vi "IncStepsESP.vi"(0 "ESP VISA IN":refnum<visa-resource-name>, 1 "Digitizer Settings":T9={"Digitizer delay (us) "=0.0, "rf points per line"=2048, "lines per plane"=128, "Samp Rate (Hz)"=100000000.0, "Additional dig delay (us)"=0.0, "Voltage Scale"=0.4, "Pre-Looks"=0, "Offset delay (us)"=0.0, "bits A/D"=8, "Avg Num"=1, "DigTimeOut"=5.0, "Rel Dig Delay"=0.0, "Dig Ch"=0, "LeCroyCluster"={"LeCroy Channels"=[TRUE, FALSE, FALSE, FALSE], "LC read pt offset"=0.0, "Sweep Avg"=FALSE}, "Main Digitizer"=enum."NI Digitizer", "Dig Config"=enum."Single channel", "Digitizer ID Cluster"={"Acqiris/Alazar/SP ID"=[], "NI Instr Handles"=[], "LeCroy VISA"="", "GaGe Handle"={"Handle"=0, "Sample size"=0, "Resolution"=0, "Offset"=0, "Channels"=0, "Boards"=0}, "ATS Ref"="ATS9350", "Acqiris Address"=["PCI::INSTR0"], "ADQRef"=refnum, "adq_cu_ptr"=refnum}, "Trigger Settings"={"Trig Source"=1, "Trig Coupling"=0, "Trig Slope"=0, "Level (mV)"=1500.0}, "Bulk Acq"=FALSE, "Bulk Start Indexes"=[], "Data Ref RF"=refnum, "NI ID/Channel"=[], "Total Dig CH"=1, "Xtra Ann Trig delay (us)"=10.0, "Fix Z Delay?"=FALSE, "One Way Transmission?"=FALSE, "Data Ref Log"=refnum} {"Trigger Settings"."Trig Slope" items=["Positive", "Negative"]; "Trigger Settings"."Level (mV)" format="%.2f"; "Trigger Settings"."Trig Coupling" items=["DC 1 MOhm", "AC 1 MOhm", "DC 50 Ohm", "AC 50 Ohm"]; "Trigger Settings"."Trig Source" items=["Chan 1", "External"]; "Rel Dig Delay" format="%.2f"; "DigTimeOut" format="%.2f"; "Avg Num" min=1; "Offset delay (us)" format="%.2f"; "Additional dig delay (us)" format="%.2f"; "Digitizer delay (us)" format="%.2f"}, 2 "Ann Array Params":T2={"Synth Foc?"=FALSE, "Focal Zones"=41, "Switch T/R"=0, "Trans Geometry (mm)"={"Transducer"=0, "Geo Focus"=12.0, "a (radius)"=3.0, "# of rings"=5, "kerf space "=0.1, "Center Freq"=12.0}, "Sub Ap Excite?"=FALSE, "Full Array Scan?"=FALSE, "Xmt/Rcv"={"XMIT"=[TRUE, TRUE, TRUE, TRUE, TRUE], "RCV"=[TRUE, TRUE, TRUE, TRUE, TRUE]}, "PulseSpacing (us)"=0.0, "Xmit Ring"=0, "XMIT CHS"=0, "RCV CHS"=0, "GPU?"=FALSE, "Save TIFF?"=FALSE, "downfactor"=1, "RCV 1CH"=0} {"RCV 1CH" items=["All", "1", "2", "3", "4", "5"]; "Trans Geometry (mm)"."Transducer" items=["6D 12R 40 MHz"=0, "10D 31R 20 MHz"=1, "10D 23R 20 MHz"=2, "6D 23R 40 MHz"=3, "4.5D 10.7R 40 MHz"=4, "9D 23.5R 20 MHz"=5, "9D 25.8R 20MHz"=6, "Enter"=99]; "Switch T/R" min=1 max=5 step=1}, 3 "Avg Num":i32=1, 5 "number of scans":i32=128, 7 "Motion Settings":T5={"No Motion?"=FALSE, "Motion System"=enum."NI 735x", "Motion Bd ID"=1, "Motion Profile"="SMAC1", "# Axis"=1, "Reverse Z axis?"=TRUE, "SMAC Axis"=0, "scan pair"=enum."y-(x) scan", "RT fps"=6.0, "Steps per mm"=[1000, 1000, 1000, 1000], "Motor Parameters"={"velocity ct/s"=[10000.0, 10000.0, 10000.0, 50000.0], "accel ct/s^2"=[50000.0, 50000.0, 50000.0, 200000.0]}, "One Way Scan"=FALSE, "Reverse One Way Scan"=FALSE, "Global Position (mm)"=[], "Plane"=0, "Distance between\nscan lines (um)"=0.0, "Distance between\nscan planes (um)"=0.0, "number of scan planes"=1, "Total steps in line"=0, "Xtra plane\ndistance  (um)"=100, "Xtra planes "=1, "Add Axis"=FALSE, "overshoot cts"=200, "BKPT Shift"=0, "Scan Start Time (ms)"=0, "ESP VISA"="GPIB::1::INSTR", "3rd Axis"=1, "GL Ref Out"=refnum, "Galil Address"=""} {"3rd Axis" items=["x", "y", "z", "w"]; "Xtra planes" min=1; "Xtra plane\ndistance  (um)" min=0; "Distance between\nscan planes (um)" format="%.2f"; "Distance between\nscan lines (um)" format="%.2f"; "SMAC Axis" items=["None"=0, "Axis 1"=1, "Axis 2"=2, "Axis 3"=3, "Axis 4"=4, "Axis 5"=5, "Axis 6"=6, "Axis 7"=7, "Axis 8"=8, "Vector Space 1"=17, "Vector Space 2"=18, "Vector Space 3"=19, "Vector Space 4"=20]; "Motion Bd ID" min=1 max=32 step=1}, 9 "Axis":i32=1 min=1 max=4, 11 "File Names":string[](array[string]), 12 "motion error in":errorcluster, 13 "Type of scan":T1, 14 "Reverse ?":bool) -> (4 "ESP VISA OUT":refnum<visa-resource-name>, 15 "Motion error":bool)   [LabVIEW 2022 SP3]
uses:
  Digitizers/-DigitizerRoutines/DigitizerSettings.ctl
  Digitizers/-DigitizerRoutines/Digitizer.ctl
  Digitizers/-DigitizerRoutines/DigConfig.ctl
  Digitizers/-DigitizerRoutines/DigitizerID.ctl
  C:/Windows/System32/ADQAPI_dotNet_helper.dll
  NI_controller/-NI_MotionRoutines/MotionParameters.ctl
  NI_controller/-NI_MotionRoutines/MotionSys.ctl
  -MotionRoutines/ScanAxis.ctl
  -MotionRoutines/3rdAxis.ctl
  Annular Array/-AnnularRoutines/AnnularArray.ctl
  Annular Array/-AnnularRoutines/TransGeometry.ctl
  Annular Array/-AnnularRoutines/ArrayGeometry.ctl
  -ScanSystem/Controls/ScanType2.ctl
  Galil/Command Menu.ctl
  <vilib>/Analysis/baseanly.llb/Mean (DBL).vi
  -MotionRoutines/MotionGlobals.vi
  <instrlib>/Acqiris Dx/Acqiris Dx.lvlib
  <instrlib>/Newport ESP301/Newport ESP301.lvlib
  <vilib>/Analysis/NI_AALBase.lvlib
panel:
  out "Intensity Graph":i16[][](graph)
  in  "Acq error in":errorcluster
  # "1-D and 2-D B scan settings"
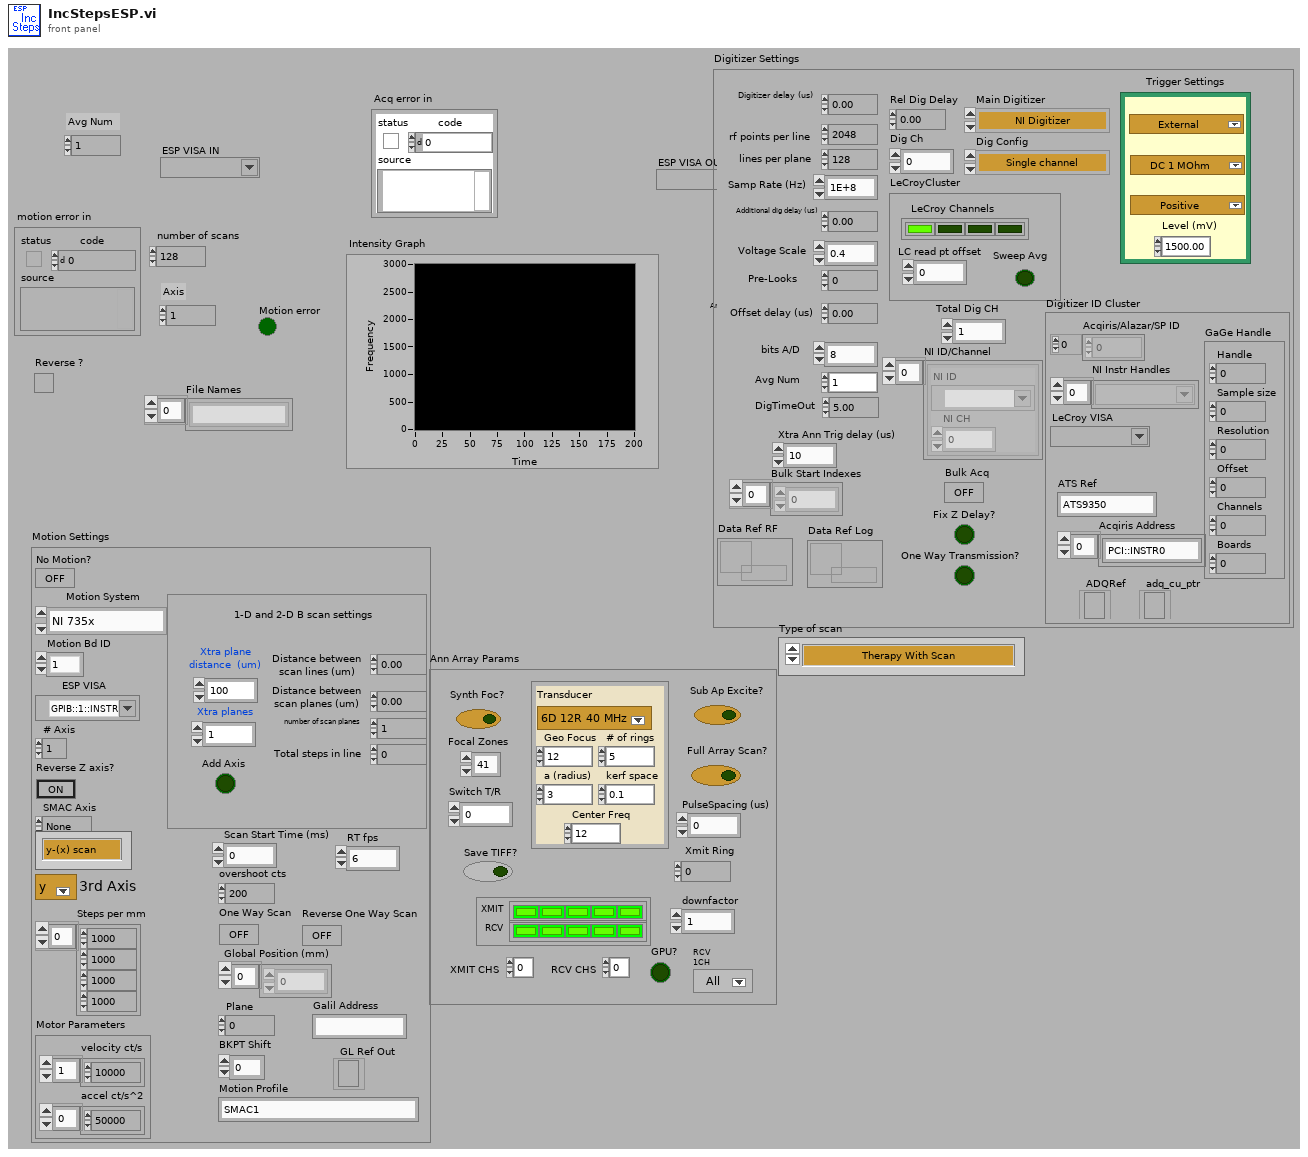
[diagram p1: front panel]
types:
  T1 = typedef "ScanType2.ctl" = enum16{"Therapy With Scan", "M scan", "M Scan With Therapy Burst", "1-D B Scan", "1-D B Scan With Therapy Burst", "2-D B Scan", "2-D B Scan With Therapy Burst", "Rotational Scan", "1-D B-Scan PRF", "2-D B-Scan PRF", "Real-Time Scan", "Contrast Agents", "1-D w/ Real-Time Set Up", "Dual Transducer", "Acoustic Microscopy", "Hydrophone Scanning"}
  T2 = typedef "AnnularArray.ctl" = cluster{"Synth Foc?":bool, "Focal Zones":i16, "Switch T/R":i16, "Trans Geometry (mm)":T3, "Sub Ap Excite?":bool, "Full Array Scan?":bool, "Xmt/Rcv":cluster{"XMIT":bool[], "RCV":bool[]}, "PulseSpacing (us)":sgl, "Xmit Ring":i32, "XMIT CHS":u8, "RCV CHS":u8, "GPU?":bool, "Save TIFF?":bool, "downfactor":i32, "RCV 1CH":u16}
  T3 = typedef "TransGeometry.ctl" = cluster{"Transducer":T4, "Geo Focus":dbl, "a (radius)":dbl, "# of rings":i32, "kerf space ":dbl, "Center Freq":dbl}
  T4 = typedef "ArrayGeometry.ctl" = u16
  T5 = typedef "MotionParameters.ctl" = cluster{"No Motion?":bool, "Motion System":T6, "Motion Bd ID":u8, "Motion Profile":string, "# Axis":i8, "Reverse Z axis?":bool, "SMAC Axis":u16, "scan pair":T7, "RT fps":sgl, "Steps per mm":i32[], "Motor Parameters":cluster{"velocity ct/s":dbl[], "accel ct/s^2":dbl[]}, "One Way Scan":bool, "Reverse One Way Scan":bool, "Global Position (mm)":dbl[], "Plane":i32, "Distance between\nscan lines (um)":sgl, "Distance between\nscan planes (um)":sgl, "number of scan planes":i32, "Total steps in line":i32, "Xtra plane\ndistance  (um)":i32, "Xtra planes ":i32, "Add Axis":bool, "overshoot cts":i32, "BKPT Shift":i32, "Scan Start Time (ms)":u32, "ESP VISA":refnum<visa-resource-name>, "3rd Axis":T8, "GL Ref Out":refnum<k7>, "Galil Address":string}
  T6 = typedef "MotionSys.ctl" = enum16{"MM3000", "NI 735x", "Newport ESP", "No Motion Card", "Galil"}
  T7 = typedef "ScanAxis.ctl" = enum16{"y-(x) scan", "x-(y) scan", "z-(x) scan", "z-(y) scan", "y-(z) scan", "x-(z) scan", "w-(x) scan", "w-(y) scan", "w-(z) scan", "x-(w) scan", "y-(w) scan", "z-(w) scan"}
  T8 = typedef "3rdAxis.ctl" = u16
  T9 = typedef "DigitizerSettings.ctl" = cluster{"Digitizer delay (us) ":dbl, "rf points per line":i32, "lines per plane":i32, "Samp Rate (Hz)":dbl, "Additional dig delay (us)":dbl, "Voltage Scale":dbl, "Pre-Looks":i32, "Offset delay (us)":dbl, "bits A/D":i8, "Avg Num":i32, "DigTimeOut":sgl, "Rel Dig Delay":sgl, "Dig Ch":i32, "LeCroyCluster":cluster{"LeCroy Channels":bool[], "LC read pt offset":dbl, "Sweep Avg":bool}, "Main Digitizer":T10, "Dig Config":T11, "Digitizer ID Cluster":T12, "Trigger Settings":cluster{"Trig Source":u16, "Trig Coupling":u16, "Trig Slope":u16, "Level (mV)":dbl}, "Bulk Acq":bool, "Bulk Start Indexes":i32[], "Data Ref RF":refnum<data-value>, "NI ID/Channel":cluster{"NI ID":refnum<k15>, "NI CH":i32}[], "Total Dig CH":i32, "Xtra Ann Trig delay (us)":dbl, "Fix Z Delay?":bool, "One Way Transmission?":bool, "Data Ref Log":refnum<data-value>}
  T10 = typedef "Digitizer.ctl" = enum16{"Acqiris Digitizer", "NI Digitizer", "LeCroy", "GaGe", "AlazarTech", "No Digitizer", "Teledyne"}
  T11 = typedef "DigConfig.ctl" = enum16{"Single channel", "2 Chans w/ 2 Acqiris", "2 Chans w/ 1 Acqiris", "5-CH Pulser New", "5-CH pulser w/ ann array", "5-pass style ann array", "Empty"}
  T12 = typedef "DigitizerID.ctl" = cluster{"Acqiris/Alazar/SP ID":u32[], "NI Instr Handles":refnum<k15>[], "LeCroy VISA":refnum<visa-resource-name>, "GaGe Handle":cluster{"Handle":u32, "Sample size":u32, "Resolution":i32, "Offset":i32, "Channels":u32, "Boards":u32}, "ATS Ref":string, "Acqiris Address":string[], "ADQRef":refnum<k24>, "adq_cu_ptr":refnum<k24>}
  T13 = typedef "location.ctl" = enum16{"Automatic", "WCM Main", "Hawaii", "Columbia MM3000", "Columbia  NI System", "NYU", "RRI 2", "UHI Allen", "CUMC RT", "Chiba", "Stony Brook", "WCM Microscopy", "WCM Aeoretch", "WCM Optics Lab", "WCM Main 2Axis", "WCM Rotation", "WCM SAM SMAC", "SERI GP"}
  T14 = typedef "Command Menu.ctl" = enum16{"CommandPassThrough", "Abort Motion", "Define Pos", "Velocity", "Acceleration", "Deceleration", "Position Rel", "Postion Abs", "Begin Move", "After Move", "Home", "KI", "KD", "KP", "IL", "Config I/O", "Set Bit", "Clear Bit", "Motor Off", "Moto On", "Status", "Execute", "Halt Execute", "HX Status", "Tell Velocity", "Check Motion", "BreakPoint", "Tell Position", "Current Code Line", "Tell Switches", "OC Force On", "OC Off", "Pos Soft Limit", "Rev Soft Limit"}
  T15 = cluster{"axis 1 +hardware travel limit":bool, "axis 2 +hardware travel limit ":bool, "axis 3 +hardware travel limit ":bool, "axis 4 +hardware travel limit ":bool, "axis 5 +hardware travel limit ":bool, "axis 6 +hardware travel limit ":bool, "reserved":bool, "reserved":bool, "axis 1 -hardware travel limit ":bool, "axis 2 -hardware travel limit ":bool, "axis 3 -hardware travel limit ":bool, "axis 4 -hardware travel limit ":bool, "axis 5 -hardware travel limit ":bool, "axis 6 -hardware travel limit ":bool, "reserved":bool, "reserved":bool, "axis 1 amplifier fault input":bool, "axis 2 amplifier fault input":bool, "axis 3 amplifier fault input":bool, "axis 4 amplifier fault input":bool, "axis 5 amplifier fault input":bool, "axis 6 amplifier fault input":bool, "reserved":bool, "reserved":bool, "reserved":bool, "reserved":bool, "reserved":bool, "100-pin emergency stop (unlatched) low":bool, "auxiliary I/O emergency stop (latched)":bool, "100-pin connector emergency stop (latched)":bool, "auxiliary I/O connector emergency stop (latched)":bool, "100-pin cable interlock":bool}
  T16 = cluster{"Port A bit-0 at logic level":bool, "Port A bit-1 at logic level":bool, "Port A bit-2 at logic level ":bool, "Port A bit-3 at logic level":bool, "Port A bit-4 at logic level":bool, "Port A bit-5 at logic level ":bool, "Port A bit-6 at logic level ":bool, "Port A bit-7 at logic level ":bool, "Port B bit-0 at logic level":bool, "Port B bit-1 at logic level":bool, "Port B bit-2 at logic level ":bool, "Port B bit-3 at logic level":bool, "Port B bit-4 at logic level":bool, "Port B bit-5 at logic level ":bool, "Port B bit-6 at logic level ":bool, "Port B bit-7 at logic level ":bool}
  T17 = cluster{sgl, "Gain [dB]  ":sgl, "Atten (dB)":sgl}[]
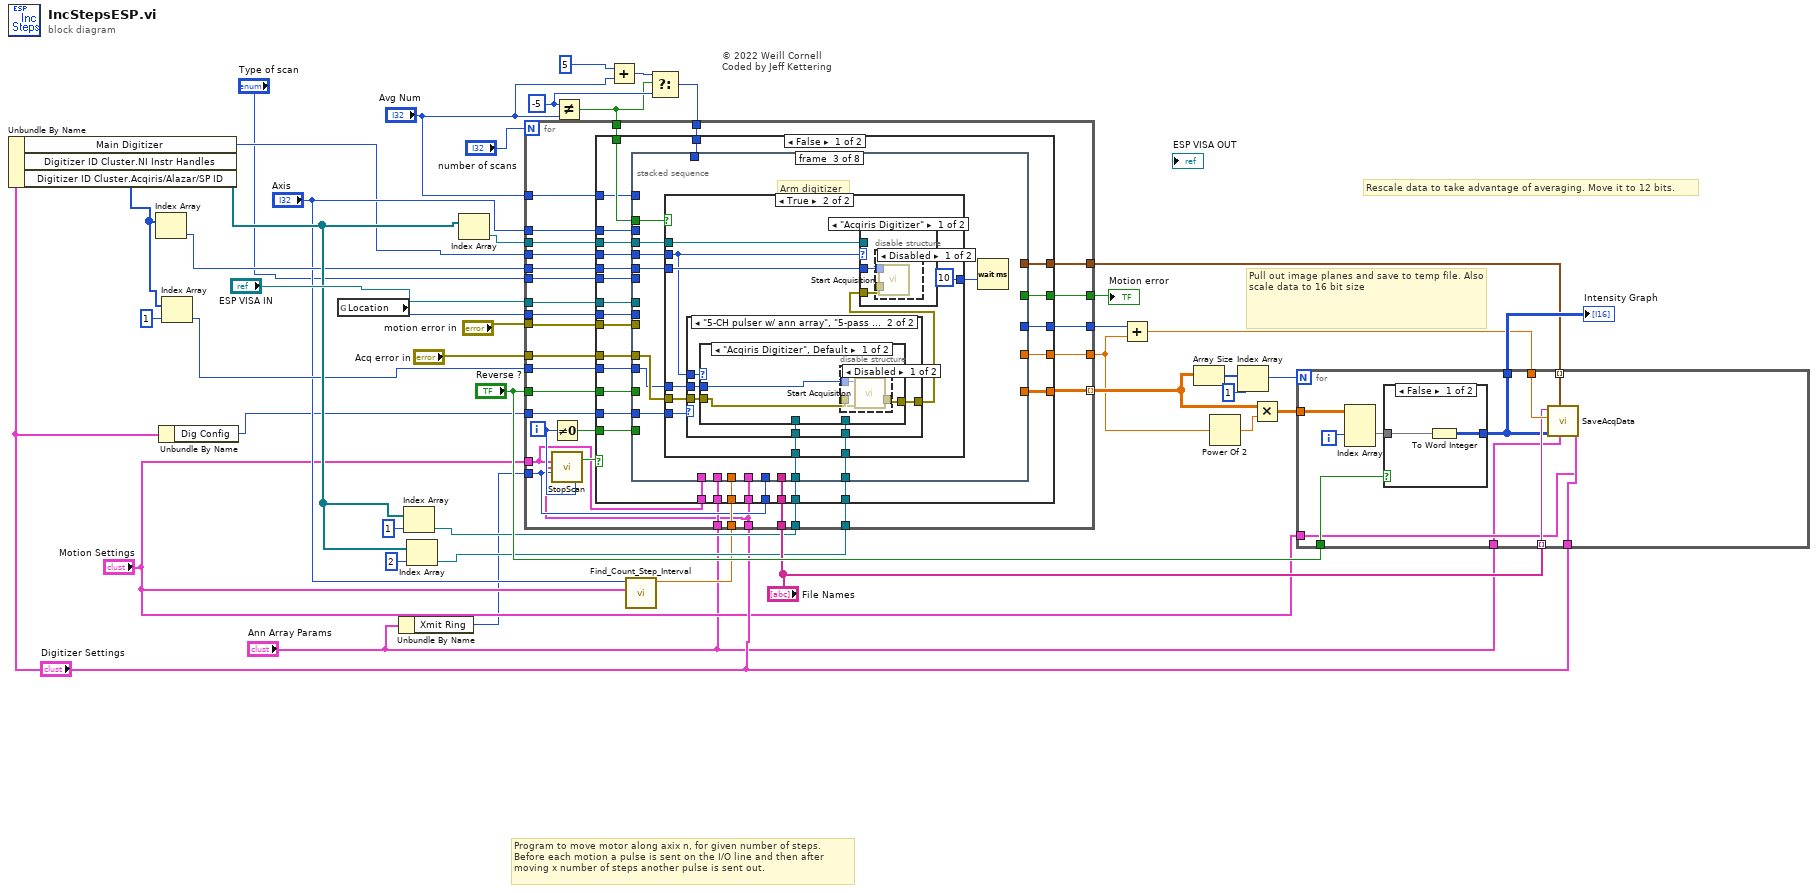
[diagram p0: block diagram]
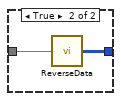
[diagram p2: hidden frame]
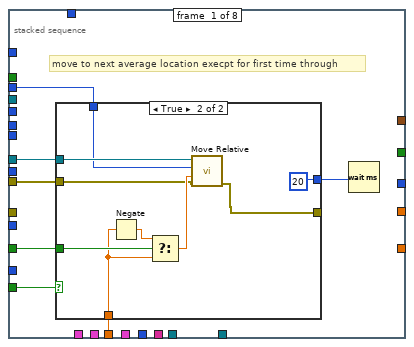
[diagram p3: hidden frame]
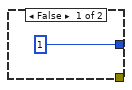
[diagram p4: hidden frame]
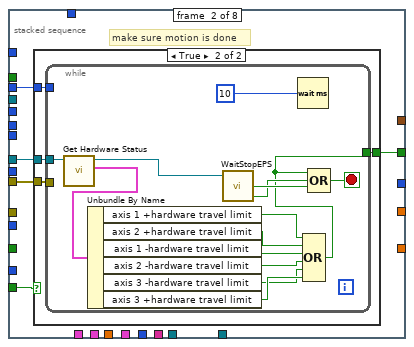
[diagram p5: hidden frame]
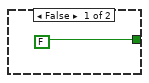
[diagram p6: hidden frame]
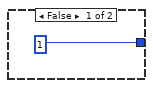
[diagram p7: hidden frame]
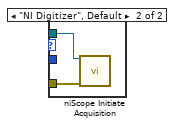
[diagram p9: hidden frame]
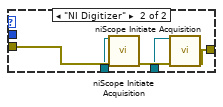
[diagram p12: hidden frame]
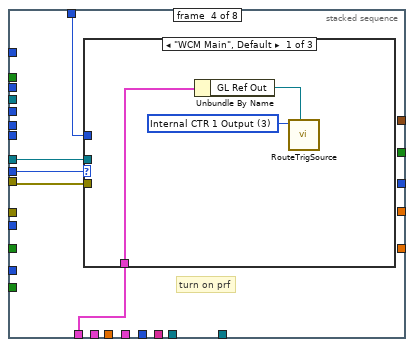
[diagram p13: hidden frame]
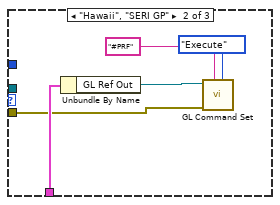
[diagram p14: hidden frame]
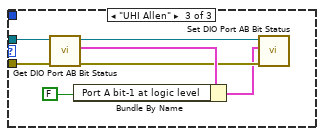
[diagram p15: hidden frame]
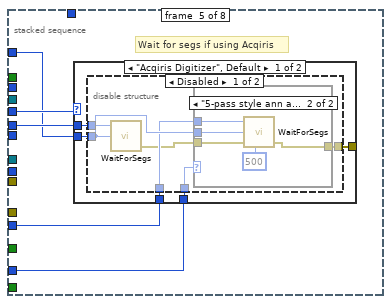
[diagram p16: hidden frame]
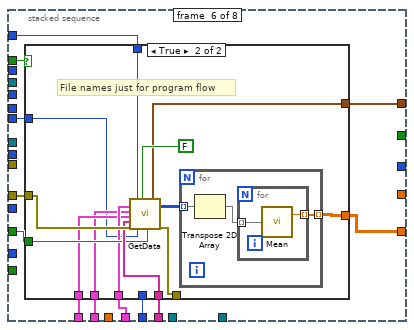
[diagram p20: hidden frame]
diagram:
  w36 = -5
  # "© 2022 Weill Cornell\nCoded by Jeff Kettering"
  # "Pull out image planes and save to temp file. Also scale data to 16 bit size"
  # "Rescale data to take advantage of averaging. Move it to 12 bits."
  # "Program to move motor along axix n, for given number of steps.\nBefore each motion a pulse is sent on the I/O line and then after\nmoving x number of steps another pulse is sent out."
  n1 = Unbundle By Name("Digitizer Settings") -> ("Main Digitizer"=w7:T10, "Digitizer ID Cluster.NI Instr Handles"=w14:refnum<k15>[], "Digitizer ID Cluster.Acqiris/Alazar/SP ID"=w11:u32[])
  n2 = Index Array(array=w11) -> (element=w13:u32)  [unwired: 1 in]
  n3 = Unbundle By Name("Digitizer Settings") -> ("Dig Config"=w5:T11)
  n4 = Index Array(array=w11, index=1) -> (element=w10:u32)
  n5 = global read "MotionGlobals.vi" "Location"() -> (w27:T13)
  n6 = Unbundle By Name("Ann Array Params") -> ("Xmit Ring"=w2:i32)
  n7 = Index Array(array=w14, index=1) -> (element=w16:refnum<k15>)
  n8 = Index Array(array=w14, index=2) -> (element=w15:refnum<k15>)
  n9 = Index Array(array=w14) -> (element=w19:refnum<k15>)  [unwired: 1 in]
  n10 = Not Equal?(x=w36, y="Avg Num") -> (x != y?=w33:bool)
  n11 = Add(x=5, y="Avg Num") -> (x+y=w34:i32)
  n12 = call "Find_Count_Step_Interval.vi"("Motion Settings In"="Motion Settings", "Axis"="Axis") -> ("BP Interval"=w8:dbl)  [unwired: 8 in, 1 out]
  n13 = Select(t=w34, s=w33, f=w36) -> (s? t:f=w37:i32)
  n14 = for {
    N: "number of scans" -> [_]
    tunnel: "ESP VISA IN" -> [w75]
    tunnel: "motion error in" -> [w74]
    tunnel: "Axis" -> [w73]
    tunnel: [w69] -> w43
    tunnel: "Reverse ?" -> [w72]
    tunnel: w37 -> [w71]
    tunnel: w13 -> [w70]
    tunnel: "Acq error in" -> [w68]
    tunnel: w5 -> [w67]
    tunnel: [w64] -> w29 mode=indexing
    tunnel: w33 -> [w66]
    tunnel: [w63] -> w23
    tunnel: w10 -> [w61]
    tunnel: "Avg Num" -> [w60]
    tunnel: w2 -> [w54]
    tunnel: w8 -> [w58]
    tunnel: w7 -> [w57]
    tunnel: w19 -> [w56]
    tunnel: w27 -> [w55]
    tunnel: [w53] -> w21
    tunnel: "File Names" -> [w52]
    tunnel: [w51] -> w24
    tunnel: w16 -> [w50]
    tunnel: w15 -> [w49]
    tunnel: "Digitizer Settings" -> [w45]
    tunnel: "Motion Settings" -> [w48]
    tunnel: "Ann Array Params" -> [w47]
    tunnel: "Type of scan" -> [w46]
    i -> [w59]
    n15 = Not Equal To 0?(x=w59) -> (x != 0?=w65:bool)
    n16 = call "StopScan.vi"("Motion Settings In"=w48, "Ring"=w54, "Digitizer Settings"=w45, "Line Number"=w59) -> ("Stop Now? Dup"=w62:bool)  [unwired: 2 in]
    n17 = case shown="False" w62 {
      tunnel: w75 -> [w104 _]
      tunnel: w74 -> [w103 _]
      tunnel: w73 -> [w102 _]
      tunnel: w72 -> [w101 _]
      tunnel: w71 -> [w100 _]
      tunnel: w70 -> [w99 _]
      tunnel: [w98 FALSE] -> w69
      tunnel: w68 -> [w97 _]
      tunnel: w67 -> [w96 _]
      tunnel: w66 -> [w95 _]
      tunnel: w65 -> [w94 _]
      tunnel: [w93 dbl[][] [] ("Data")] -> w64
      tunnel: [w92 0] -> w63
      tunnel: w61 -> [w91 _]
      tunnel: w60 -> [w90 _]
      tunnel: w58 -> [w89 _]
      tunnel: w57 -> [w88 _]
      tunnel: w56 -> [w87 _]
      tunnel: w55 -> [w86 _]
      tunnel: w54 -> [w85 _]
      tunnel: [w84 _] -> w53
      tunnel: w52 -> [w83 _]
      tunnel: [w82 _] -> w51
      tunnel: w50 -> [w81 _]
      tunnel: w49 -> [w80 _]
      tunnel: w45 -> [w79 _]
      tunnel: w48 -> [w78 _]
      tunnel: w47 -> [w77 _]
      tunnel: w46 -> [w76 _]
      frame False {
        n18 = stacked-sequence {
          tunnel: w104 -> [w111 w126 _ w194 _ _ _ _]
          tunnel: w103 -> [w110 w125 _ w193 _ _ _ _]
          tunnel: w102 -> [w109 w124 _ _ _ _ _ _]
          tunnel: [_ w123 _ _ _ _ _ _] -> w98
          tunnel: w101 -> [w108 _ _ _ _ w235 _ _]
          tunnel: w100 -> [_ _ _ w192 _ _ _ _]
          tunnel: w99 -> [_ _ w155 _ w214 _ _ _]
          tunnel: w97 -> [_ _ w149 _ _ w238 _ _]
          tunnel: w96 -> [_ _ w152 _ w210 _ _ _]
          tunnel: [_ _ _ _ _ w239 _ _] -> w93
          tunnel: w95 -> [_ _ w154 _ _ w242 _ _]
          tunnel: w94 -> [w107 w122 _ _ _ _ _ _]
          tunnel: [_ _ _ _ _ _ _ w264] -> w92
          tunnel: w91 -> [_ _ w146 _ w211 _ _ _]
          tunnel: w90 -> [_ _ _ _ w212 w241 _ w271]
          tunnel: w89 -> [w105 _ _ _ _ _ _ _]
          tunnel: w88 -> [_ _ w151 _ w213 _ _ _]
          tunnel: w87 -> [_ _ w150 _ _ _ _ _]
          tunnel: w86 -> [_ _ _ w191 _ _ w261 _]
          tunnel: w85 -> [_ _ _ _ _ w240 _ _]
          tunnel: [_ _ _ _ _ _ _ w267] -> w84
          tunnel: w83 -> [_ _ _ _ _ w237 _ _]
          tunnel: [_ _ _ _ _ w236 _ _] -> w82
          tunnel: w81 -> [_ _ w148 _ _ _ _ _]
          tunnel: w80 -> [_ _ w147 _ _ _ _ _]
          tunnel: w79 -> [_ _ _ _ _ w234 _ w263]
          tunnel: w78 -> [_ _ _ w190 _ w233 w262 _]
          tunnel: w77 -> [_ _ _ _ _ w232 _ _]
          tunnel: w76 -> [_ _ _ _ _ w231 _ _]
          frame #0 {
            # "move to next average location execpt for first time through"
            n19 = case shown="True" w107 {
              tunnel: w111 -> [_ w117]
              tunnel: w110 -> [_ w114]
              tunnel: w109 -> [_ w116]
              tunnel: w108 -> [_ w121]
              tunnel: [1 20] -> w106
              tunnel: [_ w113] -> _
              tunnel: w105 -> [_ w118]
              frame False {
              }
              frame True {
                n20 = Negate(x=w118) -> (-x=w120:dbl)
                n21 = Select(t=w120, s=w121, f=w118) -> (s? t:f=w115:dbl)
                n22 = call <instrlib>:"Move Relative.vi"("error in (no error)"=w114, "Position (0 units)"=w115, "Axis (1)"=w116, "VISA resource name"=w117) -> ("error out"=w113:errorcluster)  [unwired: 2 in, 1 out]
              }
            }
            n23 = Wait (ms)(milliseconds to wait=w106) -> ()  [unwired: 1 out]
          }
          frame #1 {
            # "make sure motion is done"
            n24 = case shown="True" w122 {
              tunnel: w126 -> [_ w131]
              tunnel: w125 -> [_ w130]
              tunnel: w124 -> [_ w129]
              tunnel: [FALSE w128] -> w123
              frame False {
              }
              frame True {
                n25 = while {
                  tunnel: w131 -> [w141]
                  tunnel: w130 -> [_]
                  tunnel: w129 -> [_]
                  tunnel: [w135] -> w128
                  stop <- w144 stop-if-true
                  n26 = call <instrlib>:"Get Hardware Status.vi"("VISA resource name"=w141) -> ("Status register 1"=w140:T15, "VISA resource name out"=w134:refnum<visa-resource-name>)  [unwired: 3 in, 2 out]
                  n27 = Unbundle By Name(w140) -> ("axis 1 +hardware travel limit"=w139:bool, "axis 2 +hardware travel limit"=w138:bool, "axis 1 -hardware travel limit"=w137:bool, "axis 2 -hardware travel limit"=w136:bool, "axis 3 -hardware travel limit"=w132:bool, "axis 3 +hardware travel limit"=w133:bool)
                  n28 = call "WaitStopEPS.vi"("VISA resource name"=w134) -> ("Error Status"=w142:bool, "Stopped"=w143:bool)  [unwired: 2 in, 1 out]
                  n29 = Wait (ms)(milliseconds to wait=10) -> ()  [unwired: 1 out]
                  n30 = Compound Arithmetic op=OR(w139, w138, w137, w136, w132, w133) -> (w135:bool)
                  n31 = Compound Arithmetic op=OR(w135, w142, w143) -> (w144:bool)
                }
              }
            }
          }
          frame #2 {
            # "Arm digitizer"
            n32 = case shown="True" w154 {
              tunnel: w155 -> [_ w166]
              tunnel: [1 10] -> w153
              tunnel: w152 -> [_ w164]
              tunnel: w151 -> [_ w162]
              tunnel: w150 -> [_ w163]
              tunnel: w149 -> [_ w161]
              tunnel: w148 -> [_ w159]
              tunnel: w147 -> [_ w158]
              tunnel: w146 -> [_ w157]
              frame False {
              }
              frame True {
                n33 = case shown="\"5-CH pulser w/ ann array\", \"5-pass style ann array\"" w164 {
                  tunnel: w162 -> [_ w178]
                  tunnel: [_ w177] -> w160
                  tunnel: w161 -> [_ w176]
                  tunnel: w159 -> [_ w175]
                  tunnel: w158 -> [_ w174]
                  tunnel: w157 -> [_ w173]
                  frame "Single channel", Default {
                  }
                  frame "5-CH pulser w/ ann array", "5-pass style ann array" {
                    n34 = case shown="\"Acqiris Digitizer\", Default" w178 {
                      tunnel: [w181 w188] -> w177
                      tunnel: w176 -> [w180 w187]
                      tunnel: w175 -> [_ w186]
                      tunnel: w174 -> [_ w185]
                      tunnel: w173 -> [w179 _]
                      frame "Acqiris Digitizer", Default {
                        n35 = disable-structure shown="Disabled" {
                          disable-tunnel: [w184 _] -> w181
                          disable-tunnel: w180 -> [w183 _]
                          disable-tunnel: w179 -> [w182 _]
                          frame Disabled {
                            n36 = call <instrlib>:"Start Acquisition.vi"("error in (no error)"=w183, "Instrument ID"=w182) -> ("error out"=w184:errorcluster)  [unwired: 2 in, 1 out]
                          }
                          frame Enabled {
                          }
                        }
                      }
                      frame "NI Digitizer" {
                        n37 = call <instrlib>:"niScope Initiate Acquisition.vi"("instrument handle"=w186, "error in"=w187) -> ("error out"=w189:errorcluster)  [unwired: 13 out]
                        n38 = call <instrlib>:"niScope Initiate Acquisition.vi"("instrument handle"=w185, "error in"=w189) -> ("error out"=w188:errorcluster)  [unwired: 13 out]
                      }
                    }
                  }
                }
                n39 = case shown="\"Acqiris Digitizer\"" w162 {
                  tunnel: w166 -> [w168 _]
                  tunnel: w163 -> [_ w172]
                  tunnel: w160 -> [w167 w171]
                  frame "Acqiris Digitizer" {
                    n40 = disable-structure shown="Disabled" {
                      disable-tunnel: w168 -> [w170 _]
                      disable-tunnel: w167 -> [w169 _]
                      frame Disabled {
                        n41 = call <instrlib>:"Start Acquisition.vi"("error in (no error)"=w169, "Instrument ID"=w170) -> ()  [unwired: 2 in, 2 out]
                      }
                      frame Enabled {
                      }
                    }
                  }
                  frame "NI Digitizer", Default {
                    n42 = call <instrlib>:"niScope Initiate Acquisition.vi"("instrument handle"=w172, "error in"=w171) -> ()  [unwired: 14 out]
                  }
                }
              }
            }
            n43 = Wait (ms)(milliseconds to wait=w153) -> ()  [unwired: 1 out]
          }
          frame #3 {
            # "turn on prf"
            n44 = case shown="\"WCM Main\", Default" w191 {
              tunnel: w194 -> [_ _ w209]
              tunnel: w193 -> [_ w198 w208]
              tunnel: w192 -> [_ _ _]
              tunnel: w190 -> [w196 w201 _]
              frame "WCM Main", Default {
                w197 = u16 3 items=["Function Gen Input", "Motion Trig", "Internal RT Motion Trig", "Internal CTR 1 Output"] ("Trig Source")
                n45 = Unbundle By Name(w196) -> ("GL Ref Out"=w195:refnum<k7>)
                n46 = call "RouteTrigSource.vi"("Galil.IGalil"=w195, "Trig Source"=w197) -> ()  [unwired: 9 in, 1 out]
              }
              frame "Hawaii", "SERI GP" {
                n47 = Unbundle By Name(w201) -> ("GL Ref Out"=w200:refnum<k7>)
                n48 = call "GL Command Set.vi"("Command"=Command_Menu."Execute", "Text Input"="#PRF", "error in (no error)"=w198, "Galil.IGalil"=w200) -> ()  [unwired: 3 in, 5 out]
              }
              frame "UHI Allen" {
                n49 = call <instrlib>:"Get DIO Port AB Bit Status.vi"("error in (no error)"=w208, "VISA resource name"=w209) -> ("error out"=w204:errorcluster, "DIO Port A status"=w207:T16, "VISA resource name out"=w205:refnum<visa-resource-name>)  [unwired: 3 in]
                n50 = Bundle By Name(cluster=w207, "Port A bit-1 at logic level"=FALSE) -> (w203:T16)
                n51 = call <instrlib>:"Set DIO Port AB Bit Status.vi"("error in (no error)"=w204, "DIO Port status"=w203, "VISA resource name"=w205) -> ()  [unwired: 3 in, 2 out]
              }
            }
          }
          frame #4 {
            # "Wait for segs if using Acqiris"
            n52 = case shown="\"Acqiris Digitizer\", Default" w213 {
              tunnel: w212 -> [w218 _]
              tunnel: w214 -> [w219 _]
              tunnel: [w215 _] -> _
              tunnel: w211 -> [w217 _]
              tunnel: w210 -> [w216 _]
              frame "Acqiris Digitizer", Default {
                n53 = disable-structure shown="Disabled" {
                  disable-tunnel: w219 -> [w225 _]
                  disable-tunnel: w218 -> [w224 _]
                  disable-tunnel: w217 -> [w223 _]
                  disable-tunnel: w216 -> [w222 _]
                  disable-tunnel: [w220 _] -> w215
                  frame Disabled {
                    n54 = call "WaitForSegs.vi"("Acqiris ID"=w225, "lines per plane"=w224) -> ("error out"=w221:errorcluster)  [unwired: 2 in, 3 out]
                    n55 = case shown="\"5-pass style ann array\"" w222 {
                      tunnel: w223 -> [_ w230]
                      tunnel: w224 -> [_ w228]
                      tunnel: w221 -> [_ w227]
                      tunnel: [_ w226] -> w220
                      frame "Single channel", Default {
                      }
                      frame "5-pass style ann array" {
                        n56 = call "WaitForSegs.vi"("Acqiris ID"=w230, "lines per plane"=w228, "error in"=w227, "Timeout"=500) -> ("error out"=w226:errorcluster)  [unwired: 3 out]
                      }
                    }
                  }
                  frame Enabled {
                  }
                }
              }
              frame "NI Digitizer" {
              }
            }
          }
          frame #5 {
            n57 = case shown="True" w242 {
              tunnel: w241 -> [_ w254]
              tunnel: w240 -> [_ _]
              tunnel: [_ w252] -> w239
              tunnel: w238 -> [_ w251]
              tunnel: w237 -> [_ w250]
              tunnel: [_ w249] -> _
              tunnel: [_ w248] -> w236
              tunnel: w235 -> [_ w247]
              tunnel: w234 -> [_ w246]
              tunnel: w233 -> [_ w245]
              tunnel: w232 -> [_ w244]
              tunnel: w231 -> [_ w243]
              frame False {
              }
              frame True {
                # "File names just for program flow"
                n58 = call "GetData.vi"("Digitizer Settings"=w246, "Ann Array Params"=w244, "Motion Settings"=w245, "All files"=w250, "error in"=w251, "lines per plane mod"=w254, "Type of scan"=w243, "save?"=FALSE, "Reverse ?"=w247) -> ("Gain Array"=w248:T17, "Raw data out"=w253:i16[][][], "error out"=w249:errorcluster)  [unwired: 8 in]
                n59 = for {
                  tunnel: w253 -> [w258] mode=indexing
                  tunnel: [w256] -> w252 mode=indexing
                  n60 = Transpose 2D Array(2D array=w258) -> (transposed array=w257:i16[][])
                  n61 = for {
                    tunnel: w257 -> [w260] mode=indexing
                    tunnel: [w259] -> w256 mode=indexing
                    n62 = call-poly <vilib>:"Mean.vi"("X"=w260) -> ("mean"=w259:dbl)  [unwired: 1 out]
                  }
                }
              }
            }
          }
          frame #6 {
            # "turn off prf"
            n63 = call "PRF_Off.vi"("Location"=w261, "Motion Settings In"=w262) -> ()  [unwired: 9 in, 1 out]
          }
          frame #7 {
            # "choose bits for final save format"
            n64 = Unbundle By Name(w263) -> ("bits A/D"=w264:i8)
            n65 = Logarithm Base 2(1:w271) -> (0:w270:dbl)
            n66 = Round Toward +Infinity(x=w270) -> (ceil(x): smallest int >= x=w269:dbl)
            n67 = Subtract(x=16, y=w264) -> (x-y=w265:i32)
            n68 = In Range and Coerce(upper limit=w265, x=w269, lower limit=0.0) -> (coerced(x)=w267:dbl)  [unwired: 1 out]
          }
        }
      }
      frame True {
      }
    }
  }
  "Motion error" <- w43
  n69 = Add(x=w23, y=w21) -> (x+y=w22:dbl)
  n70 = Array Size(array=w29) -> (size(s)=w40:i32[])
  n71 = Power Of 2(x=w21) -> (2^x=w30:dbl)
  n72 = Index Array(array=w40, index=1) -> (element=w38:i32)
  n73 = Multiply(x=w29, y=w30) -> (x*y=w28:dbl[][][])
  n74 = for {
    N: w38 -> [_]
    tunnel: w28 -> [w285]
    tunnel: "Reverse ?" -> [w283]
    tunnel: w22 -> [w282]
    tunnel: "File Names" -> [w280] mode=indexing
    tunnel: [w279] -> w26
    tunnel: w24 -> [w278] mode=indexing
    tunnel: "Digitizer Settings" -> [w277]
    tunnel: "Motion Settings" -> [w276]
    tunnel: "Ann Array Params" -> [w275]
    i -> [w284]
    n75 = Index Array(array=w285, index (dim 1)=w284) -> (element=w281:dbl[][])  [unwired: 2 in]
    n76 = case shown="False" w283 {
      tunnel: w281 -> [w287 w289]
      tunnel: [w286 w288] -> w279
      frame False {
        n77 = To Word Integer(number=w287) -> (16bit integer=w286:i16[][])
      }
      frame True {
        n78 = call "ReverseData.vi"("Array in"=w289) -> ("Array out"=w288:i16[][])
      }
    }
    n79 = call "SaveAcqData.vi"("Digitizer Settings"=w277, "Motion Settings"=w276, "Ann Array Params"=w275, "Votage scaling"=w278, "Array"=w279, "Dig Word Size"=w282, "File Name"=w280) -> ()  [unwired: 4 in]
  }
  "Intensity Graph" <- w26
